vi "LoadPalpationWrapper-Kamronn-Medtech.vi"(8 "error in":errorcluster, 11 "File dir":path) -> (0 "error out":errorcluster, 3 "palpation":cluster{"right":string, "left":string})   [LabVIEW 2013, in "main.lvlib"]
uses:
  main.lvlib
  <userlib>/_OpenG.lib/file/file.llb/File Exists - Scalar__ogtk.vi
  Globals/DataPathGlobalVariable.vi
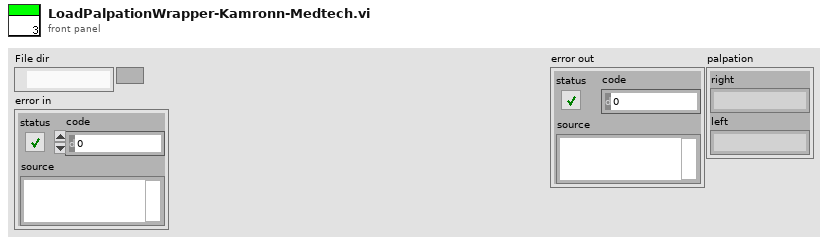
[diagram p1: front panel]
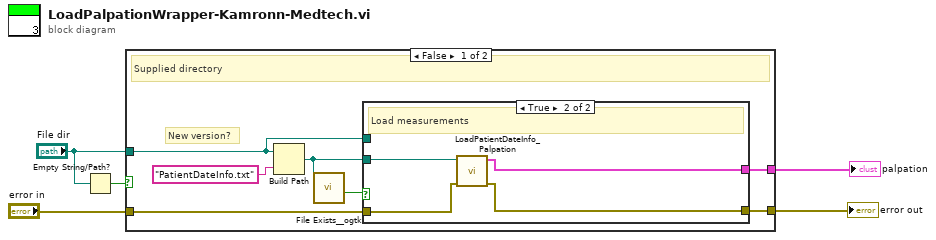
[diagram p0: block diagram]
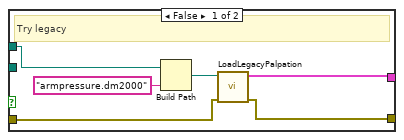
[diagram p2: hidden frame]
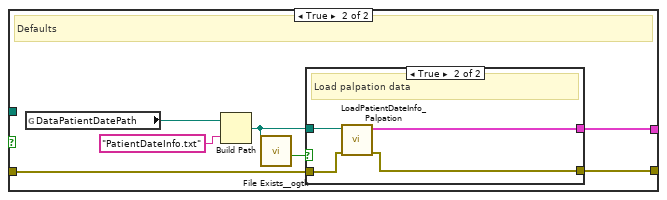
[diagram p3: hidden frame]
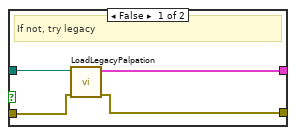
[diagram p4: hidden frame]
diagram:
  n1 = Empty String/Path?(string/path="File dir") -> (empty?=w5:bool)
  n2 = case shown="False" w5 {
    tunnel: "File dir" -> [w7 _]
    tunnel: "error in" -> [w9 w25]
    tunnel: [w8 w24] -> w2
    tunnel: [w6 w23] -> w1
    frame False {
      # "New version?"
      # "Supplied directory"
      n3 = Build Path(base path=w7, name or relative path="PatientDateInfo.txt") -> (appended path=w10:path)
      n4 = call-poly <userlib>:"File Exists__ogtk.vi"("file path"=w10) -> ("exists"=w11:bool)  [unwired: 6 in, 1 out]
      n5 = case shown="True" w11 {
        tunnel: w10 -> [_ w22]
        tunnel: w9 -> [w16 w21]
        tunnel: [w15 w20] -> w8
        tunnel: w7 -> [w14 _]
        tunnel: [w13 w19] -> w6
        frame False {
          # "Try legacy"
          n6 = Build Path(base path=w14, name or relative path="armpressure.dm2000") -> (appended path=w17:path)
          n7 = call "LoadLegacyPalpation.vi"("error in (no error)"=w16, "File path"=w17) -> ("error out"=w15:errorcluster, "Palpation"=w13:cluster{"Right":string, "Left":string})  [unwired: 8 in]
        }
        frame True {
          # "Load measurements"
          n8 = call "LoadPatientDateInfo_Palpation.vi"("error in"=w21, "File path"=w22) -> ("error out"=w20:errorcluster, "palpation"=w19:cluster{"right":string, "left":string})  [unwired: 8 in]
        }
      }
    }
    frame True {
      # "Defaults"
      n9 = global read "DataPathGlobalVariable.vi" "DataPatientDatePath"() -> (w28:path)
      n10 = Build Path(base path=w28, name or relative path="PatientDateInfo.txt") -> (appended path=w26:path)
      n11 = call-poly <userlib>:"File Exists__ogtk.vi"("file path"=w26) -> ("exists"=w27:bool)  [unwired: 6 in, 1 out]
      n12 = case shown="True" w27 {
        tunnel: w26 -> [w33 w37]
        tunnel: w25 -> [w31 w36]
        tunnel: [w32 w35] -> w24
        tunnel: [w30 w34] -> w23
        frame False {
          # "If not, try legacy"
          n13 = call "LoadLegacyPalpation.vi"("error in (no error)"=w31, "File path"=w33) -> ("error out"=w32:errorcluster, "Palpation"=w30:cluster{"Right":string, "Left":string})  [unwired: 8 in]
        }
        frame True {
          # "Load palpation data"
          n14 = call "LoadPatientDateInfo_Palpation.vi"("error in"=w36, "File path"=w37) -> ("error out"=w35:errorcluster, "palpation"=w34:cluster{"right":string, "left":string})  [unwired: 8 in]
        }
      }
    }
  }
  "error out" <- w2
  "palpation" <- w1
